vi "Run Service.vi"() -> ()   [LabVIEW 2021, in "streamtest_server.lvlib"]
uses:
  streamtest_server.lvlib
  RPC Messages/streamtest_StreamData.ctl
  <vilib>/gRPC/LabVIEW gRPC Servicer/Servicer/Servicer.lvclass/Servicer.ctl
  RPC Service/stream/stream.lvclass
  C:/Program Files/National Instruments/LabVIEW 2021/vi.lib/gRPC/LabVIEW gRPC Servicer/ServiceBase/ServiceBase.lvclass
  RPC Service/stream/stream.lvclass/stream.ctl
  <vilib>/gRPC/LabVIEW gRPC Servicer/Servicer/Servicer.lvclass
panel:
  in  "milliseconds to wait":u32=1
  in  "stop":bool
  in  "Numeric":i32=2000
  out "output cluster":T1
  out "error out 2":errorcluster
  out "Listening Port":i32
  in  "Stop":bool
  in  "Server Address":string="localhost:50051"
  in  "Server Certificate File (.crt)":path
  in  "Server Key File (.key)":path
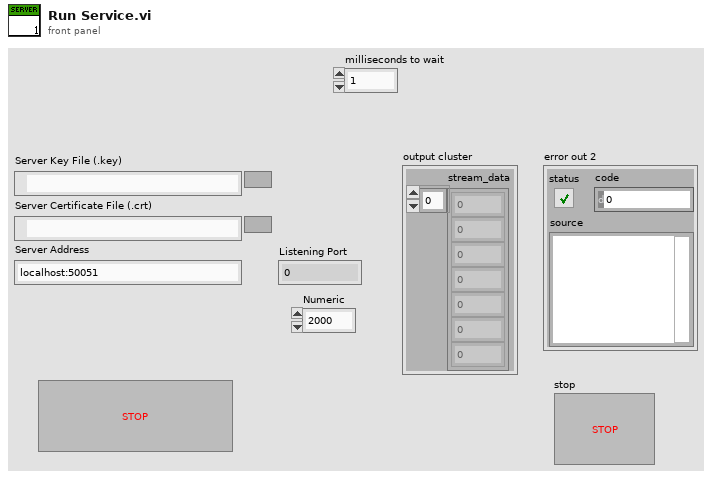
[diagram p1: front panel]
types:
  T1 = typedef "streamtest_server.lvlib/streamtest_StreamData.ctl" = cluster{"stream_data":u8[]}
  T2 = typedef "grpc-lvsupport-release.lvlib/grpcId.ctl" = u64
  T3 = typedef "streamtest_server.lvlib/stream.lvclass/Server Internal UEs.ctl" = cluster{"stream Send Internal UE":refnum<user-event>}
  T4 = typedef "streamtest_server.lvlib/stream.lvclass/Server gRPC UEs.ctl" = cluster{"stream Send gRPC UE":refnum<user-event>}
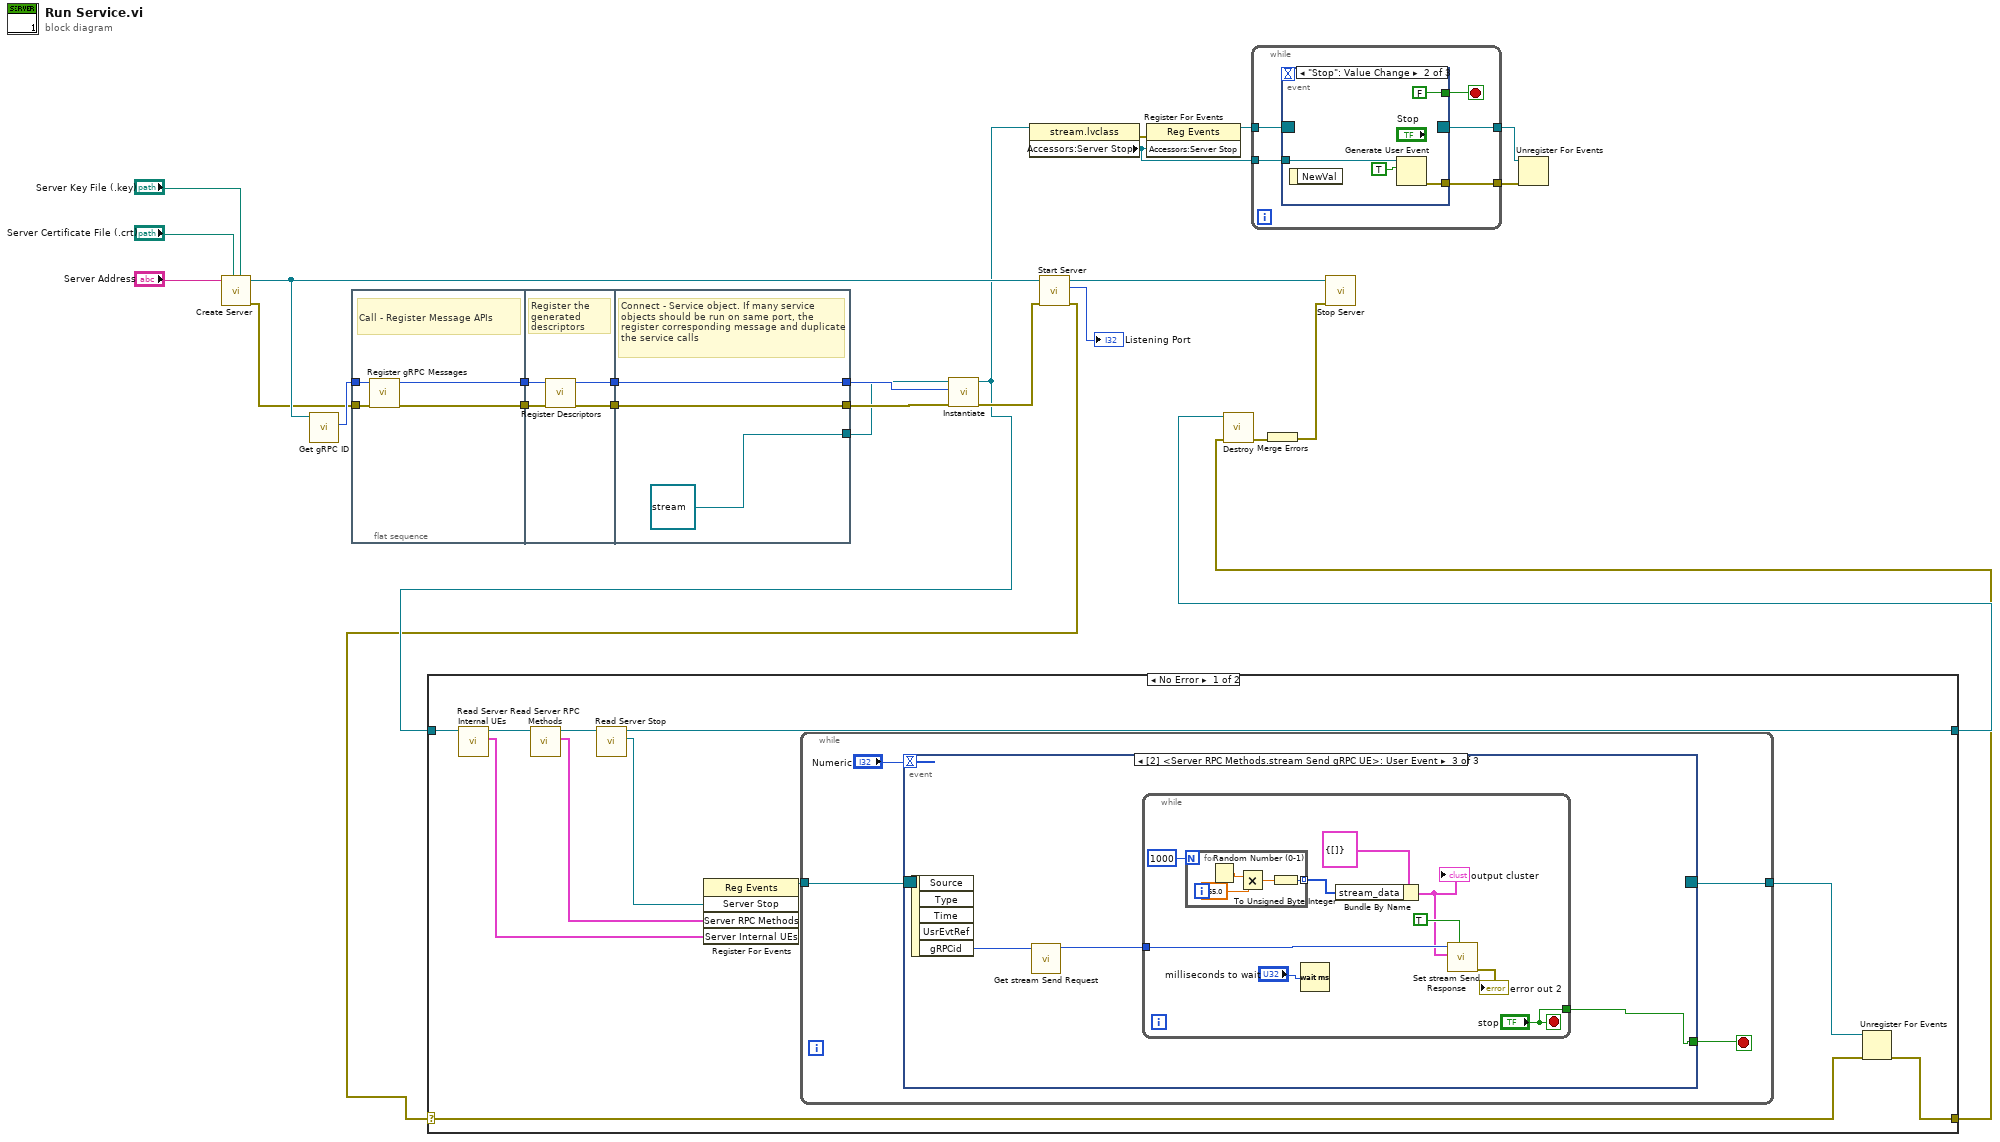
[diagram p0: block diagram]
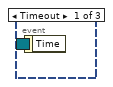
[diagram p2: hidden frame]
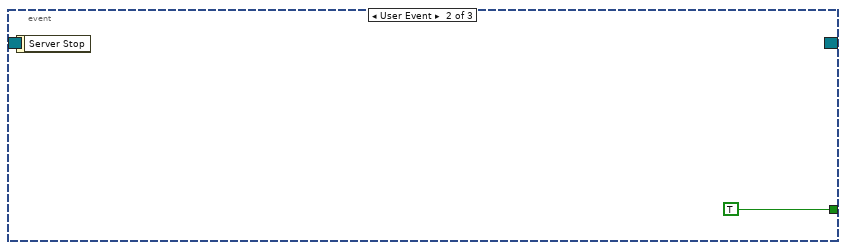
[diagram p3: hidden frame]
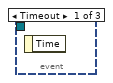
[diagram p5: hidden frame]
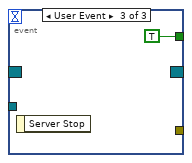
[diagram p6: hidden frame]
diagram:
  n1 = call <vilib>:"Create Server.vi"("Server Key File (.key)"="Server Key File (.key)", "Server Certificate File (.crt)"="Server Certificate File (.crt)", "Server Address"="Server Address") -> ("error out"=w13:errorcluster, "gRPC Server out"=w20:refnum<class "Servicer.lvclass">)  [unwired: 7 in]
  n2 = call <vilib>:"Get gRPC ID.vi"("OOP Server in"=w20) -> ("gRPC ID"=w14:T2)  [unwired: 9 in, 1 out]
  n3 = flat-sequence {
    tunnel: w14 -> [w29]
    tunnel: w13 -> [w31]
    tunnel: [w30] -> w9
    tunnel: [w28] -> w8
    tunnel: w9 -> [w34]
    tunnel: w8 -> [w35]
    tunnel: [w32] -> w7
    tunnel: [w33] -> w6
    tunnel: [w37] -> w11
    tunnel: [w38] -> w12
    tunnel: w7 -> [w38]
    tunnel: w6 -> [w37]
    tunnel: [refnum<class "stream.lvclass"> refnum ("streamtest_server.lvlib:stream.lvclass")] -> w5
    frame #0 {
      # "Call - Register Message APIs"
      n4 = call "Register gRPC Messages.vi"("error in (no error)"=w31, "gRPC ID"=w29) -> ("error out"=w30:errorcluster, "gRPC ID Out"=w28:T2)  [unwired: 8 in]
    }
    frame #1 {
      # "Register the generated descriptors"
      n5 = call "Register Descriptors.vi"("error in (no error)"=w34, "gRPC ID"=w35) -> ("error out"=w32:errorcluster, "gRPC ID Out"=w33:T2)  [unwired: 8 in]
    }
    frame #2 {
      # "Connect - Service object. If many service objects should be run on same port, the register corresponding message and duplicate the service calls"
    }
  }
  n6 = call-dynamic "Instantiate.vi"("error in"=w12, "gRPCid"=w11, "iService"=w5) -> ("error out"=w18:errorcluster, "iService"=w4:refnum<class "stream.lvclass">)  [unwired: 7 in]
  n7 = property class="stream.lvclass"(reference=w4) -> (error out=w19:errorcluster, "Accessors:Server Stop"=w10:refnum<user-event>)  [unwired: 1 in, 1 out]
  n8 = call <vilib>:"Start Server.vi"("error in"=w18, "gRPC Server in"=w20) -> ("error out"=w3:errorcluster, "Listening Port"=→"Listening Port":i32, "gRPC Server out"=w27:refnum<class "Servicer.lvclass">)  [unwired: 7 in]
  n9 = case shown="No Error" w3 {
    selector: w3 -> [w43 w72]
    tunnel: [w42 w72] -> w1
    tunnel: [w40 w71] -> w2
    tunnel: w4 -> [w49 w71]
    frame No Error {
      n10 = call "Read Server Internal UEs.vi"("SignalGeneratorService in"=w49) -> ("Server Internal UEs"=w47:T3, "SignalGeneratorService out"=w48:refnum<class "stream.lvclass">)  [unwired: 8 in, 1 out]
      n11 = call "Read Server RPC Methods.vi"("SignalGeneratorService in"=w48) -> ("Server RPC Methods"=w41:T4, "SignalGeneratorService out"=w46:refnum<class "stream.lvclass">)  [unwired: 8 in, 1 out]
      n12 = call-dynamic "Read Server Stop.vi"("iService in"=w46) -> ("Server Stop"=w39:refnum<user-event>, "iService out"=w40:refnum<class "stream.lvclass">)  [unwired: 8 in, 1 out]
      n13 = register-events(w39, w41, w47) -> (reference out=w45:refnum<event-registration>)  [unwired: 2 in, 1 out]
      n14 = while {
        tunnel: w45 -> [w53]
        tunnel: [w51] -> w44
        stop <- w52 stop-if-true
        n15 = event "RPC Methods Event Structure" shown="[2] <Server RPC Methods.stream Send gRPC UE>: User Event" {
          selector: w53 -> [_ _ _]
          dyn-events: [_ _ _] -> w51
          timeout: "Numeric" -> [_ _ _]
          tunnel: [_ TRUE w55] -> w52
          event Timeout {
            n16 = event-data() -> ()  [unwired: 1 in, 1 out]
          }
          event User Event {
            n17 = event-data() -> ()  [unwired: 1 in, 1 out]
          }
          event User Event {
            n18 = event-data() -> ("gRPCid"=w57:T2)  [unwired: 1 in, 4 out]
            n19 = call "Get stream Send Request.vi"("gRPCid"=w57) -> ("gRPCid out"=w56:T2)  [unwired: 8 in, 2 out]
            n20 = while {
              tunnel: w56 -> [w66]
              tunnel: ["stop"] -> w55
              stop <- "stop" stop-if-true
              n21 = for {
                N: 1000 -> [_]
                tunnel: [w67] -> w62 mode=indexing
                n22 = Random Number (0-1)() -> (number: 0 to 1=w70:dbl)
                n23 = Multiply(x=w70, y=255.0) -> (x*y=w68:dbl)
                n24 = To Unsigned Byte Integer(number=w68) -> (unsigned 8bit integer=w67:u8)
              }
              n25 = Wait (ms)(milliseconds to wait="milliseconds to wait") -> ()  [unwired: 1 out]
              n26 = Bundle By Name(cluster=T1 {"stream_data"=[]} ("Message Data"), "stream_data"=w62) -> (w61:T1)
              "output cluster" <- w61
              n27 = call "Set stream Send Response.vi"("Streaming? (F)"=TRUE, "Message Data"=w61, "gRPCid in"=w66) -> ("error out"=→"error out 2":errorcluster)  [unwired: 8 in]
            }
          }
        }
      }
      n28 = Unregister For Events(event registration refnum=w44, error in=w43) -> (error out=w42:errorcluster)
    }
    frame Error {
    }
  }
  n29 = register-events(error in=w19, w10) -> (reference out=w23:refnum<event-registration>)  [unwired: 1 in, 1 out]
  n30 = call-dynamic "Destroy.vi"("error in (no error)"=w1, "SignalGeneratorService in"=w2) -> ("error out"=w17:errorcluster)  [unwired: 8 in, 1 out]
  n31 = while {
    tunnel: w23 -> [w77]
    tunnel: [w75] -> w22
    tunnel: [w73] -> w15
    tunnel: w10 -> [w74]
    stop <- w76 stop-if-true
    n32 = event shown="[1] \"Stop\": Value Change" {
      selector: w77 -> [_ _ _]
      dyn-events: [_ _ _] -> w75
      timeout: _ -> [_ _ _]
      tunnel: [_ FALSE TRUE] -> w76
      tunnel: w74 -> [_ w80 _]
      tunnel: [_ w78 _] -> w73
      event Timeout {
        n33 = event-data() -> ()  [unwired: 1 in, 1 out]
      }
      event "Stop": Value Change {
        n34 = event-data() -> ()  [unwired: 1 in, 1 out]
        n35 = Generate User Event(user event=w80, event data cluster=TRUE ("event data")) -> (error out=w78:errorcluster)  [unwired: 2 in, 1 out]
      }
      event User Event {
        n36 = event-data() -> ()  [unwired: 1 in, 1 out]
      }
    }
  }
  n37 = Merge Errors(w17) -> (w16:errorcluster)
  n38 = call <vilib>:"Stop Server.vi"("error in"=w16, "gRPC Server in"=w27) -> ()  [unwired: 9 in, 1 out]
  n39 = Unregister For Events(event registration refnum=w22, error in=w15) -> ()  [unwired: 1 out]
